vi "CAEN_HVBoard.ProcEvents.vi"(0 "i ref in":refnum<vi>, 5 "error in":errorcluster) -> (14 "i ref out":refnum<vi>, 19 "error out":errorcluster)   [LabVIEW 2014, in "CAEN_HVBoard.lvlib"]
doc: "This method is used to define the events the object will listen to. Add your own events here."
uses:
  CAEN_HVBoard.lvlib
  CSCore/BaseProcess/BaseProcess.event definition.ctl
  CSCore/CAEObj/CAEObj.event definition.ctl
  CSCore/BaseProcess/BaseProcess.descriptor string definition.ctl
  CSCore/BaseProcess/BaseProcess.lvlib
  CSCore/CAEObj/CAEObj.lvlib
panel:
  in  "event definition":T1={"CAEEvtDef"={"URL"="lvmsg://setKill", "enable"=TRUE, "ignoreResID"=FALSE}, "Data Descriptor"="S:1 n[Kill] //If Kill=True: Switch OFF at the max rate all system channels;"}
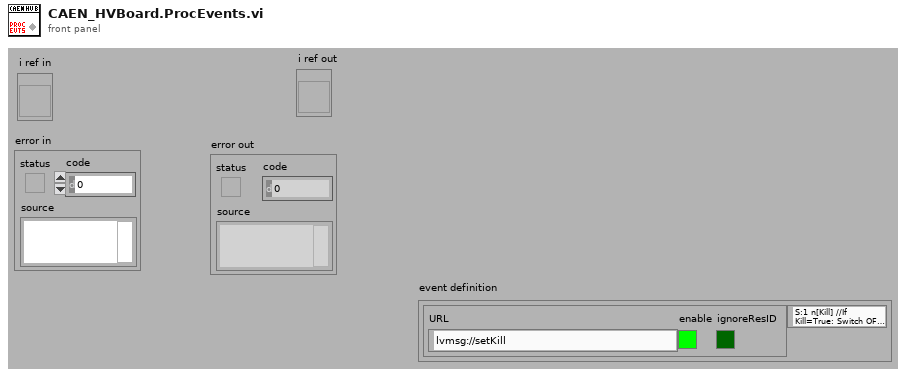
[diagram p1: front panel]
types:
  T1 = typedef "BaseProcess.lvlib/BaseProcess.event definition.ctl" = cluster{"CAEEvtDef":T2, "Data Descriptor":T3}
  T2 = typedef "CAEObj.lvlib/CAEObj.event definition.ctl" = cluster{"URL":string, "enable":bool, "ignoreResID":bool}
  T3 = typedef "BaseProcess.lvlib/BaseProcess.descriptor string definition.ctl" = string
  T4 = typedef "CAEN_HVBoard.lvlib/CAEN_HVBoard.i attribute.ctl" = cluster{"System Name":string, "Board ID":i32, "Prefix":string, "HVMaxMultiplier":dbl, "Temp#Multiplier":dbl, "Model Name":cluster{"Model Name":string, "DIM Status":cluster{"no link":bool, "quality":i32, "Time Stamp":timestamp}}, "Description":cluster{"Description":string, "DIM Status":cluster{"no link":bool, "quality":i32, "Time Stamp":timestamp}}, "SerNum":cluster{"SerNum":i16, "DIM Status":cluster{"no link":bool, "quality":i32, "Time Stamp":timestamp}}, "NrOfCh":cluster{"NrOfCh":i16, "DIM Status":cluster{"no link":bool, "quality":i32, "Time Stamp":timestamp}}, "BdStatus":cluster{"BdStatus":i16, "DIM Status":cluster{"no link":bool, "quality":i32, "Time Stamp":timestamp}}, "HVMax":cluster{"HVMax":dbl, "DIM Status":cluster{"no link":bool, "quality":i32, "Time Stamp":timestamp}}, "HVMax#EU":cluster{"HVMax#EU":string, "DIM Status":cluster{"no link":bool, "quality":i32, "Time Stamp":timestamp}}, "HVMax#HighEU":cluster{"HVMax#HighEU":dbl, "DIM Status":cluster{"no link":bool, "quality":i32, "Time Stamp":timestamp}}, "HVMax#LowEU":cluster{"HVMax#LowEU":dbl, "DIM Status":cluster{"no link":bool, "quality":i32, "Time Stamp":timestamp}}, "Temp#EU":cluster{"Temp#EU":string, "DIM Status":cluster{"no link":bool, "quality":i32, "Time Stamp":timestamp}}, "Temp":cluster{"Temp":dbl, "DIM Status":cluster{"no link":bool, "quality":i32, "Time Stamp":timestamp}}, "Temp#HighEU":cluster{"Temp#HighEU":dbl, "DIM Status":cluster{"no link":bool, "quality":i32, "Time Stamp":timestamp}}, "Temp#LowEU":cluster{"Temp#LowEU":dbl, "DIM Status":cluster{"no link":bool, "quality":i32, "Time Stamp":timestamp}}}
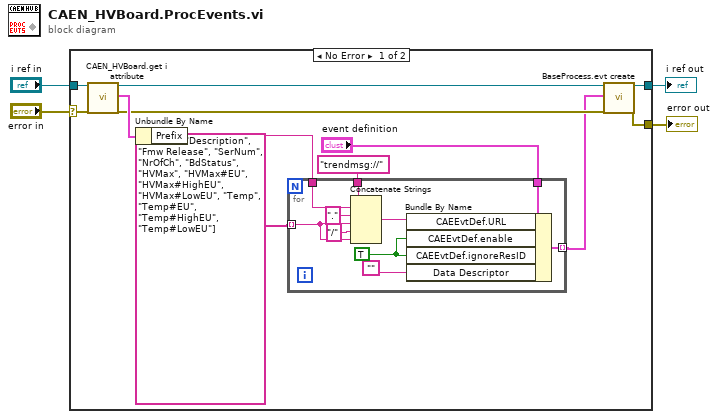
[diagram p0: block diagram]
diagram:
  n1 = case shown="No Error" "error in" {
    selector: "error in" -> [w7 w27]
    tunnel: "i ref in" -> [w9 w28]
    tunnel: [w16 w28] -> w3
    tunnel: [w15 w27] -> w2
    frame No Error {
      n2 = call "CAEN_HVBoard.get i attribute.vi"("i ref in"=w9, "error in (no error)"=w7) -> ("i ref out"=w8:refnum<vi>, "i attribute"=w11:T4, "error out"=w6:errorcluster)  [unwired: 15 in]
      n3 = Unbundle By Name(w11) -> ("Prefix"=w10:string)
      n4 = for {
        tunnel: "event definition" -> [w26]
        tunnel: "trendmsg://" -> [w25]
        tunnel: string[] ["Model", "Description", "Fmw Release", "SerNum", "NrOfCh", "BdStatus", "HVMax", "HVMax#EU", "HVMax#HighEU", "HVMax#LowEU", "Temp", "Temp#EU", "Temp#HighEU", "Temp#LowEU"] -> [w20] mode=indexing
        tunnel: [w19] -> w5 mode=indexing
        tunnel: w10 -> [w17]
        w23 = TRUE ("CAEEvtDef.ignoreResID")
        n5 = Concatenate Strings(w25, w17, "." ("string"), w20, "/" ("string"), w20) -> (w24:string)
        n6 = Bundle By Name(cluster=w26, "CAEEvtDef.URL"=w24, "CAEEvtDef.enable"=w23, "CAEEvtDef.ignoreResID"=w23, "Data Descriptor"="") -> (w19:T1)
      }
      n7 = call "BaseProcess.evt create.vi"("i ref in"=w8, "newEvents"=w5, "error in (no error)"=w6) -> ("i ref out"=w16:refnum<vi>, "error out"=w15:errorcluster)  [unwired: 13 in, 2 out]
    }
    frame Error {
    }
  }
  "i ref out" <- w3
  "error out" <- w2
